vi "Update.vi"(4 "Value2":dbl, 6 "Value1":dbl, 8 "error in (no error)":errorcluster, 9 "Audio History Buffer In":dbl[][](array[numeric]), 10 "Audio Data In":dbl[][](array[numeric]), 11 "Crusher in":refnum<class "Crusher.lvclass">) -> (0 "error out":errorcluster, 1 "Audio History Buffer Out":dbl[][](array[numeric]), 2 "Audio Data Out":dbl[][](array[numeric]), 3 "Crusher out":refnum<class "Crusher.lvclass">)   [LabVIEW 2019, in "Crusher.lvlib" / "Crusher.lvclass"]
doc: "Applies bit crusher type effects. The audio signal is reduced in both sampling frequency and bit depth, producing a harsh, digital sound.\n\n<b>Value1:</b> Sampling frequency reduction factor\n<b>Value2:</b> Bit depth (1-16)"
uses:
  Crusher.lvclass
  <vilib>/Analysis/2dsp.llb/Decimate (single shot, DBL).vi
  <vilib>/gmath/NI_Gmath.lvlib
  <vilib>/Analysis/NI_AALPro.lvlib
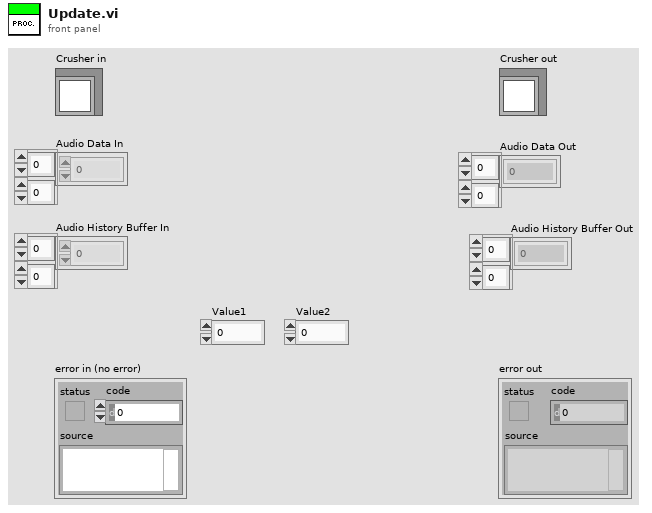
[diagram p1: front panel]
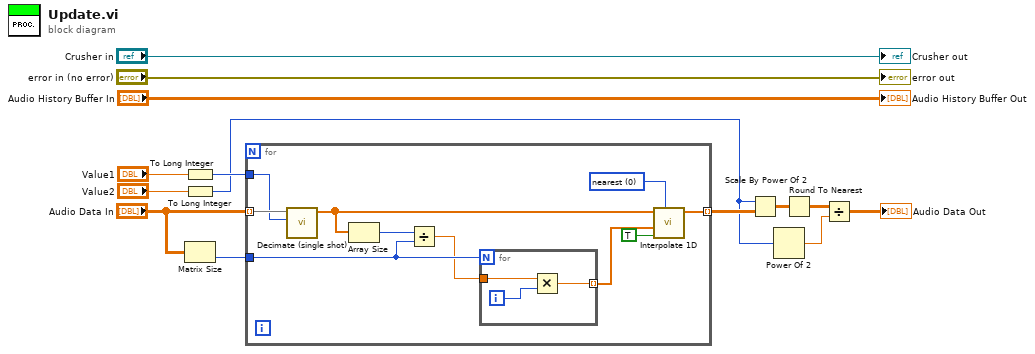
[diagram p0: block diagram]
diagram:
  n1 = To Long Integer(number="Value1") -> (32bit integer=w8:i32)
  n2 = To Long Integer(number="Value2") -> (32bit integer=w7:i32)
  n3 = Matrix Size(0:"Audio Data In") -> (2:w13:i32)  [unwired: 1 out]
  n4 = for {
    tunnel: "Audio Data In" -> [w24] mode=indexing
    tunnel: w8 -> [w23]
    tunnel: w13 -> [w21]
    tunnel: [w15] -> w12 mode=indexing
    w16 = 0 items=["nearest", "linear", "spline", "cubic Hermite", "Lagrange"] ("method")
    n5 = call-poly <vilib>:"Decimate (single shot).vi"("decimating factor"=w23, "X"=w24) -> ("Decimated Array"=w17:dbl[])  [unwired: 8 in, 1 out]
    n6 = Array Size(array=w17) -> (size(s)=w22:i32)
    n7 = Divide(x=w22, y=w21) -> (x/y=w20:dbl)
    n8 = for {
      N: w21 -> [_]
      tunnel: w20 -> [w27]
      tunnel: [w25] -> w19 mode=indexing
      i -> [w26]
      n9 = Multiply(x=w27, y=w26) -> (x*y=w25:dbl)
    }
    n10 = call <vilib>:"Interpolate 1D.vi"("method"=w16, "X is monotonic"=TRUE, "xi"=w19, "Y"=w17) -> ("yi"=w15:dbl[])  [unwired: 5 in, 2 out]
  }
  n11 = Scale By Power Of 2(n=w7, x=w12) -> (x*2^n=w11:dbl[][])
  n12 = Power Of 2(x=w7) -> (2^x=w9:dbl)
  n13 = Round To Nearest(number=w11) -> (nearest integer value=w10:dbl[][])
  n14 = Divide(x=w10, y=w9) -> (x/y=→"Audio Data Out":dbl[][])
  "error out" <- "error in (no error)"
  "Crusher out" <- "Crusher in"
  "Audio History Buffer Out" <- "Audio History Buffer In"
